vi "RangeXML_Flo.vi"() -> ()   [LabVIEW 2013]
panel:
  out "text":string
  out "LabVIEW Data 2":variant
  out "array":u16[](array[numeric])=[0, 0, 1, 1, 2, 2, 3, 3, 0, 0, 1, 1, 2, 2, 3, 3, 0, 0, 1, 1, 2, 2, 3, 3, 0, 0, 1, 1, 2, 2, 3, 3, 0, 0, 1, 1, 2, 2, 3, 3, 0, 0, 1, 1, 2, 2, 3, 3, 0, 0, 1, 1, 2, 2, 3, 3, 0, 0, 1, 1, 2, 2, 3, 3, 0, 0, 1, 1, 2, 2, 3, 3, 0, 0, 1, 1, 2, 2, 3, 3, 0, 0, 1, 1, 2, 2, 3, 3, 0, 0, 1, 1, 2, 2, 3, 3, 0, 0, 1, 1, 2, 2, 3, 3, 0, 0, 1, 1, 2, 2, 3, 3, 0, 0, 1, 1, 2, 2, 3, 3, 0, 0, 1, 1, 2, 2, 3, 3]
  in  "BoloRange_mV":T1={"Channel001"=0, "Channel002"=0, "Channel003"=1, "Channel004"=1, "Channel005"=2, "Channel006"=2, "Channel007"=3, "Channel008"=3, "Channel009"=0, "Channel010"=0, "Channel011"=1, "Channel012"=1, "Channel013"=2, "Channel014"=2, "Channel015"=3, "Channel016"=3, "Channel017"=0, "Channel018"=0, "Channel019"=1, "Channel020"=1, "Channel021"=2, "Channel022"=2, "Channel023"=3, "Channel024"=3, "Channel025"=0, "Channel026"=0, "Channel027"=1, "Channel028"=1, "Channel029"=2, "Channel030"=2, "Channel031"=3, "Channel032"=3, "Channel033"=0, "Channel034"=0, "Channel035"=1, "Channel036"=1, "Channel037"=2, "Channel038"=2, "Channel039"=3, "Channel040"=3, "Channel041"=0, "Channel042"=0, "Channel043"=1, "Channel044"=1, "Channel045"=2, "Channel046"=2, "Channel047"=3, "Channel048"=3, "Channel049"=0, "Channel050"=0, "Channel051"=1, "Channel052"=1, "Channel053"=2, "Channel054"=2, "Channel055"=3, "Channel056"=3, "Channel057"=0, "Channel058"=0, "Channel059"=1, "Channel060"=1, "Channel061"=2, "Channel062"=2, "Channel063"=3, "Channel064"=3, "Channel065"=0, "Channel066"=0, "Channel067"=1, "Channel068"=1, "Channel069"=2, "Channel070"=2, "Channel071"=3, "Channel072"=3, "Channel073"=0, "Channel074"=0, "Channel075"=1, "Channel076"=1, "Channel077"=2, "Channel078"=2, "Channel079"=3, "Channel080"=3, "Channel081"=0, "Channel082"=0, "Channel083"=1, "Channel084"=1, "Channel085"=2, "Channel086"=2, "Channel087"=3, "Channel088"=3, "Channel089"=0, "Channel090"=0, "Channel091"=1, "Channel092"=1, "Channel093"=2, "Channel094"=2, "Channel095"=3, "Channel096"=3, "Channel097"=0, "Channel098"=0, "Channel099"=1, "Channel100"=1, "Channel101"=2, "Channel102"=2, "Channel103"=3, "Channel104"=3, "Channel105"=0, "Channel106"=0, "Channel107"=1, "Channel108"=1, "Channel109"=2, "Channel110"=2, "Channel111"=3, "Channel112"=3, "Channel113"=0, "Channel114"=0, "Channel115"=1, "Channel116"=1, "Channel117"=2, "Channel118"=2, "Channel119"=3, "Channel120"=3, "Channel121"=0, "Channel122"=0, "Channel123"=1, "Channe124"=1, "Channel125"=2, "Channel126"=2, "Channel127"=3, "Channel128"=3} {"Channel128" items=["10", "20", "40", "80"]; "Channel127" items=["10", "20", "40", "80"]; "Channel126" items=["10", "20", "40", "80"]; "Channel125" items=["10", "20", "40", "80"]; "Channe124" items=["10", "20", "40", "80"]; "Channel123" items=["10", "20", "40", "80"]; "Channel122" items=["10", "20", "40", "80"]; "Channel121" items=["10", "20", "40", "80"]; "Channel120" items=["10", "20", "40", "80"]; "Channel119" items=["10", "20", "40", "80"]; "Channel118" items=["10", "20", "40", "80"]; "Channel117" items=["10", "20", "40", "80"]; "Channel116" items=["10", "20", "40", "80"]; "Channel115" items=["10", "20", "40", "80"]; "Channel114" items=["10", "20", "40", "80"]; "Channel113" items=["10", "20", "40", "80"]; "Channel112" items=["10", "20", "40", "80"]; "Channel111" items=["10", "20", "40", "80"]; "Channel110" items=["10", "20", "40", "80"]; "Channel109" items=["10", "20", "40", "80"]; "Channel108" items=["10", "20", "40", "80"]; "Channel107" items=["10", "20", "40", "80"]; "Channel106" items=["10", "20", "40", "80"]; "Channel105" items=["10", "20", "40", "80"]; "Channel104" items=["10", "20", "40", "80"]; "Channel103" items=["10", "20", "40", "80"]; "Channel102" items=["10", "20", "40", "80"]; "Channel101" items=["10", "20", "40", "80"]; "Channel100" items=["10", "20", "40", "80"]; "Channel099" items=["10", "20", "40", "80"]; "Channel098" items=["10", "20", "40", "80"]; "Channel097" items=["10", "20", "40", "80"]; "Channel096" items=["10", "20", "40", "80"]; "Channel095" items=["10", "20", "40", "80"]; "Channel094" items=["10", "20", "40", "80"]; "Channel093" items=["10", "20", "40", "80"]; "Channel092" items=["10", "20", "40", "80"]; "Channel091" items=["10", "20", "40", "80"]; "Channel090" items=["10", "20", "40", "80"]; "Channel089" items=["10", "20", "40", "80"]; "Channel088" items=["10", "20", "40", "80"]; "Channel087" items=["10", "20", "40", "80"]; "Channel086" items=["10", "20", "40", "80"]; "Channel085" items=["10", "20", "40", "80"]; "Channel084" items=["10", "20", "40", "80"]; "Channel083" items=["10", "20", "40", "80"]; "Channel082" items=["10", "20", "40", "80"]; "Channel081" items=["10", "20", "40", "80"]; "Channel080" items=["10", "20", "40", "80"]; "Channel079" items=["10", "20", "40", "80"]; "Channel078" items=["10", "20", "40", "80"]; "Channel077" items=["10", "20", "40", "80"]; "Channel076" items=["10", "20", "40", "80"]; "Channel075" items=["10", "20", "40", "80"]; "Channel074" items=["10", "20", "40", "80"]; "Channel073" items=["10", "20", "40", "80"]; "Channel072" items=["10", "20", "40", "80"]; "Channel071" items=["10", "20", "40", "80"]; "Channel070" items=["10", "20", "40", "80"]; "Channel069" items=["10", "20", "40", "80"]; "Channel068" items=["10", "20", "40", "80"]; "Channel067" items=["10", "20", "40", "80"]; "Channel066" items=["10", "20", "40", "80"]; "Channel065" items=["10", "20", "40", "80"]; "Channel064" items=["10", "20", "40", "80"]; "Channel063" items=["10", "20", "40", "80"]; "Channel062" items=["10", "20", "40", "80"]; "Channel061" items=["10", "20", "40", "80"]; "Channel060" items=["10", "20", "40", "80"]; "Channel059" items=["10", "20", "40", "80"]; "Channel058" items=["10", "20", "40", "80"]; "Channel057" items=["10", "20", "40", "80"]; "Channel056" items=["10", "20", "40", "80"]; "Channel055" items=["10", "20", "40", "80"]; "Channel054" items=["10", "20", "40", "80"]; "Channel053" items=["10", "20", "40", "80"]; "Channel052" items=["10", "20", "40", "80"]; "Channel051" items=["10", "20", "40", "80"]; "Channel050" items=["10", "20", "40", "80"]; "Channel049" items=["10", "20", "40", "80"]; "Channel048" items=["10", "20", "40", "80"]; "Channel047" items=["10", "20", "40", "80"]; "Channel046" items=["10", "20", "40", "80"]; "Channel045" items=["10", "20", "40", "80"]; "Channel044" items=["10", "20", "40", "80"]; "Channel043" items=["10", "20", "40", "80"]; "Channel042" items=["10", "20", "40", "80"]; "Channel041" items=["10", "20", "40", "80"]; "Channel040" items=["10", "20", "40", "80"]; "Channel039" items=["10", "20", "40", "80"]; "Channel038" items=["10", "20", "40", "80"]; "Channel037" items=["10", "20", "40", "80"]; "Channel036" items=["10", "20", "40", "80"]; "Channel035" items=["10", "20", "40", "80"]; "Channel034" items=["10", "20", "40", "80"]; "Channel033" items=["10", "20", "40", "80"]; "Channel032" items=["10", "20", "40", "80"]; "Channel031" items=["10", "20", "40", "80"]; "Channel030" items=["10", "20", "40", "80"]; "Channel029" items=["10", "20", "40", "80"]; "Channel028" items=["10", "20", "40", "80"]; "Channel027" items=["10", "20", "40", "80"]; "Channel026" items=["10", "20", "40", "80"]; "Channel025" items=["10", "20", "40", "80"]; "Channel024" items=["10", "20", "40", "80"]; "Channel023" items=["10", "20", "40", "80"]; "Channel022" items=["10", "20", "40", "80"]; "Channel021" items=["10", "20", "40", "80"]; "Channel020" items=["10", "20", "40", "80"]; "Channel019" items=["10", "20", "40", "80"]; "Channel018" items=["10", "20", "40", "80"]; "Channel017" items=["10", "20", "40", "80"]; "Channel016" items=["10", "20", "40", "80"]; "Channel015" items=["10", "20", "40", "80"]; "Channel014" items=["10", "20", "40", "80"]; "Channel013" items=["10", "20", "40", "80"]; "Channel012" items=["10", "20", "40", "80"]; "Channel011" items=["10", "20", "40", "80"]; "Channel010" items=["10", "20", "40", "80"]; "Channel009" items=["10", "20", "40", "80"]; "Channel008" items=["10", "20", "40", "80"]; "Channel007" items=["10", "20", "40", "80"]; "Channel006" items=["10", "20", "40", "80"]; "Channel005" items=["10", "20", "40", "80"]; "Channel004" items=["10", "20", "40", "80"]; "Channel003" items=["10", "20", "40", "80"]; "Channel002" items=["10", "20", "40", "80"]; "Channel001" items=["10", "20", "40", "80"]}
  out "LabVIEW Data":variant=variant(cluster{"Channel001":u16, "Channel002":u16, "Channel003":u16, "Channel004":u16, "Channel005":u16, "Channel006":u16, "Channel007":u16, "Channel008":u16, "Channel009":u16, "Channel010 ":u16, "Channel011":u16, "Channel012":u16, "Channel013 ":u16, "Channel014":u16, "Channel015":u16, "Channel016":u16, "Channel017":u16, "Channel018 ":u16, "Channel019":u16, "Channel020":u16, "Channel021":u16, "Channel022":u16, "Channel023":u16, "Channel024":u16, "Channel025":u16, "Channel026":u16, "Channel027":u16, "Channel028":u16, "Channel029":u16, "Channel030":u16, "Channel031":u16, "Channel032":u16, "Channel033":u16, "Channel034":u16, "Channel035":u16, "Channel036":u16, "Channel037":u16, "Channel038":u16, "Channel039":u16, "Channel040":u16, "Channel041":u16, "Channel042":u16, "Channel043 ":u16, "Channel044":u16, "Channel045 ":u16, "Channel046":u16, "Channel047":u16, "Channel048":u16, "Channel049":u16, "Channel050 ":u16, "Channel051":u16, "Channel052":u16, "Channel053":u16, "Channel054":u16, "Channel55":u16, "Channel56":u16, "Channel57":u16, "Channel58":u16, "Channel59":u16, "Channe60":u16, "Channel61":u16, "Channel62":u16, "Channe63":u16, "Channel64":u16, "Channel65":u16, "Channel66":u16, "Channel67":u16, "Channel68":u16, "Channel69":u16, "Channel70":u16, "Channel71":u16, "Channel72":u16, "Channel73":u16, "Channel74 ":u16, "Channel75":u16, "Channe76":u16, "Channel77":u16, "Channel78":u16, "Channel79":u16, "Channel80":u16, "Channel81":u16, "Channel82 ":u16, "Channel83":u16, "Channel84":u16, "Channel85":u16, "Channel86":u16, "Channel87":u16, "Channel88":u16, "Channel89":u16, "Channel90":u16, "Channel91":u16, "Channe92":u16, "Channel93":u16, "Channel94":u16, "Channe95":u16, "Channel96":u16, "Channel97":u16, "Channel98":u16, "Channel99":u16, "Channel36 2":u16, "Channel37 2":u16, "Channel38 2":u16, "Channel39 2":u16, "Channel40 2":u16, "Channel41 2":u16, "Channel42 2":u16, "Channel43  2":u16, "Channe44 2":u16, "Channel45  2":u16, "Channel46 2":u16, "Channel47 2":u16, "Channel48 2":u16, "Channel113":u16, "Channel114":u16, "Channel115":u16, "Channel116":u16, "Channel117":u16, "Channel118":u16, "Channel119":u16, "Channel120":u16, "Channel121":u16, "Channel122":u16, "Channel123":u16, "Channe124":u16, "Channel125":u16, "Channel126":u16, "Channel127":u16, "Channel128":u16} {"Channel001"=0, "Channel002"=0, "Channel003"=1, "Channel004"=1, "Channel005"=2, "Channel006"=2, "Channel007"=3, "Channel008"=3, "Channel009"=0, "Channel010 "=0, "Channel011"=1, "Channel012"=1, "Channel013 "=2, "Channel014"=2, "Channel015"=3, "Channel016"=3, "Channel017"=0, "Channel018 "=0, "Channel019"=1, "Channel020"=1, "Channel021"=2, "Channel022"=2, "Channel023"=3, "Channel024"=3, "Channel025"=0, "Channel026"=0, "Channel027"=1, "Channel028"=1, "Channel029"=2, "Channel030"=2, "Channel031"=3, "Channel032"=3, "Channel033"=0, "Channel034"=0, "Channel035"=1, "Channel036"=1, "Channel037"=2, "Channel038"=2, "Channel039"=3, "Channel040"=3, "Channel041"=0, "Channel042"=0, "Channel043 "=1, "Channel044"=1, "Channel045 "=2, "Channel046"=2, "Channel047"=3, "Channel048"=3, "Channel049"=0, "Channel050 "=0, "Channel051"=1, "Channel052"=1, "Channel053"=2, "Channel054"=2, "Channel55"=3, "Channel56"=3, "Channel57"=0, "Channel58"=0, "Channel59"=1, "Channe60"=1, "Channel61"=2, "Channel62"=2, "Channe63"=3, "Channel64"=3, "Channel65"=0, "Channel66"=0, "Channel67"=1, "Channel68"=1, "Channel69"=2, "Channel70"=2, "Channel71"=3, "Channel72"=3, "Channel73"=0, "Channel74 "=0, "Channel75"=1, "Channe76"=1, "Channel77"=2, "Channel78"=2, "Channel79"=3, "Channel80"=3, "Channel81"=0, "Channel82 "=0, "Channel83"=1, "Channel84"=1, "Channel85"=2, "Channel86"=2, "Channel87"=3, "Channel88"=3, "Channel89"=0, "Channel90"=0, "Channel91"=1, "Channe92"=1, "Channel93"=2, "Channel94"=2, "Channe95"=3, "Channel96"=3, "Channel97"=0, "Channel98"=0, "Channel99"=1, "Channel36 2"=1, "Channel37 2"=2, "Channel38 2"=2, "Channel39 2"=3, "Channel40 2"=3, "Channel41 2"=0, "Channel42 2"=0, "Channel43  2"=1, "Channe44 2"=1, "Channel45  2"=2, "Channel46 2"=2, "Channel47 2"=3, "Channel48 2"=3, "Channel113"=0, "Channel114"=0, "Channel115"=1, "Channel116"=1, "Channel117"=2, "Channel118"=2, "Channel119"=3, "Channel120"=3, "Channel121"=0, "Channel122"=0, "Channel123"=1, "Channe124"=1, "Channel125"=2, "Channel126"=2, "Channel127"=3, "Channel128"=3})
  out "XML String":string="<BoloRange_mV>\r\n  <Channel001>0</Channel001>\r\n  <Channel002>0</Channel002>\r\n  <Channel003>1</Channel003>\r\n  <Channel004>1</Channel004>\r\n  <Channel005>2</Channel005>\r\n  <Channel006>2</Channel006>\r\n  <Channel007>3</Channel007>\r\n  <Channel008>3</Channel008>\r\n  <Channel009>0</Channel009>\r\n  <Channel010_>0</Channel010_>\r\n  <Channel011>1</Channel011>\r\n  <Channel012>1</Channel012>\r\n  <Channel013_>2</Channel013_>\r\n  <Channel014>2</Channel014>\r\n  <Channel015>3</Channel015>\r\n  <Channel016>3</Channel016>\r\n  <Channel017>0</Channel017>\r\n  <Channel018_>0</Channel018_>\r\n  <Channel019>1</Channel019>\r\n  <Channel020>1</Channel020>\r\n  <Channel021>2</Channel021>\r\n  <Channel022>2</Channel022>\r\n  <Channel023>3</Channel023>\r\n  <Channel024>3</Channel024>\r\n  <Channel025>0</Channel025>\r\n  <Channel026>0</Channel026>\r\n  <Channel027>1</Channel027>\r\n  <Channel028>1</Channel028>\r\n  <Channel029>2</Channel029>\r\n  <Channel030>2</Channel030>\r\n  <Channel031>3</Channel031>\r\n  <Channel032>3</Channel032>\r\n  <Channel033>0</Channel033>\r\n  <Channel034>0</Channel034>\r\n  <Channel035>1</Channel035>\r\n  <Channel036>1</Channel036>\r\n  <Channel037>2</Channel037>\r\n  <Channel038>2</Channel038>\r\n  <Channel039>3</Channel039>\r\n  <Channel040>3</Channel040>\r\n  <Channel041>0</Channel041>\r\n  <Channel042>0</Channel042>\r\n  <Channel043_>1</Channel043_>\r\n  <Channel044>1</Channel044>\r\n  <Channel045_>2</Channel045_>\r\n  <Channel046>2</Channel046>\r\n  <Channel047>3</Channel047>\r\n  <Channel048>3</Channel048>\r\n  <Channel049>0</Channel049>\r\n  <Channel050_>0</Channel050_>\r\n  <Channel051>1</Channel051>\r\n  <Channel052>1</Channel052>\r\n  <Channel053>2</Channel053>\r\n  <Channel054>2</Channel054>\r\n  <Channel055>3</Channel055>\r\n  <Channel056>3</Channel056>\r\n  <Channel057>0</Channel057>\r\n  <Channel058>0</Channel058>\r\n  <Channel059>1</Channel059>\r\n  <Channe60>1</Channe60>\r\n  <Channel061>2</Channel061>\r\n  <Channel062>2</Channel062>\r\n  <Channe63>3</Channe63>\r\n  <Channel064>3</Channel064>\r\n  <Channel065>0</Channel065>\r\n  <Channel066>0</Channel066>\r\n  <Channel067>1</Channel067>\r\n  <Channel068>1</Channel068>\r\n  <Channel069>2</Channel069>\r\n  <Channel070>2</Channel070>\r\n  <Channel071>3</Channel071>\r\n  <Channel072>3</Channel072>\r\n  <Channel073>0</Channel073>\r\n  <Channel074_>0</Channel074_>\r\n  <Channel075>1</Channel075>\r\n  <Channe76>1</Channe76>\r\n  <Channel077>2</Channel077>\r\n  <Channel078>2</Channel078>\r\n  <Channel079>3</Channel079>\r\n  <Channel080>3</Channel080>\r\n  <Channel081>0</Channel081>\r\n  <Channel082_>0</Channel082_>\r\n  <Channel083>1</Channel083>\r\n  <Channel084>1</Channel084>\r\n  <Channel085>2</Channel085>\r\n  <Channel086>2</Channel086>\r\n  <Channel087>3</Channel087>\r\n  <Channel088>3</Channel088>\r\n  <Channel089>0</Channel089>\r\n  <Channel090>0</Channel090>\r\n  <Channel091>1</Channel091>\r\n  <Channe92>1</Channe92>\r\n  <Channel093>2</Channel093>\r\n  <Channel094>2</Channel094>\r\n  <Channe95>3</Channe95>\r\n  <Channel096>3</Channel096>\r\n  <Channel097>0</Channel097>\r\n  <Channel098>0</Channel098>\r\n  <Channel099>1</Channel099>\r\n  <Channel36_2>1</Channel36_2>\r\n  <Channel37_2>2</Channel37_2>\r\n  <Channel38_2>2</Channel38_2>\r\n  <Channel39_2>3</Channel39_2>\r\n  <Channel40_2>3</Channel40_2>\r\n  <Channel41_2>0</Channel41_2>\r\n  <Channel42_2>0</Channel42_2>\r\n  <Channel43__2>1</Channel43__2>\r\n  <Channe44_2>1</Channe44_2>\r\n  <Channel45__2>2</Channel45__2>\r\n  <Channel46_2>2</Channel46_2>\r\n  <Channel47_2>3</Channel47_2>\r\n  <Channel48_2>3</Channel48_2>\r\n  <Channel113>0</Channel113>\r\n  <Channel114>0</Channel114>\r\n  <Channel115>1</Channel115>\r\n  <Channel116>1</Channel116>\r\n  <Channel117>2</Channel117>\r\n  <Channel118>2</Channel118>\r\n  <Channel119>3</Channel119>\r\n  <Channel120>3</Channel120>\r\n  <Channel121>0</Channel121>\r\n  <Channel122>0</Channel122>\r\n  <Channel123>1</Channel123>\r\n  <Channe124>1</Channe124>\r\n  <Channel125>2</Channel125>\r\n  <Channel126>2</Channel126>\r\n  <Channel127>3</Channel127>\r\n  <Channel128>3</Channel128>\r\n</BoloRange_mV>"
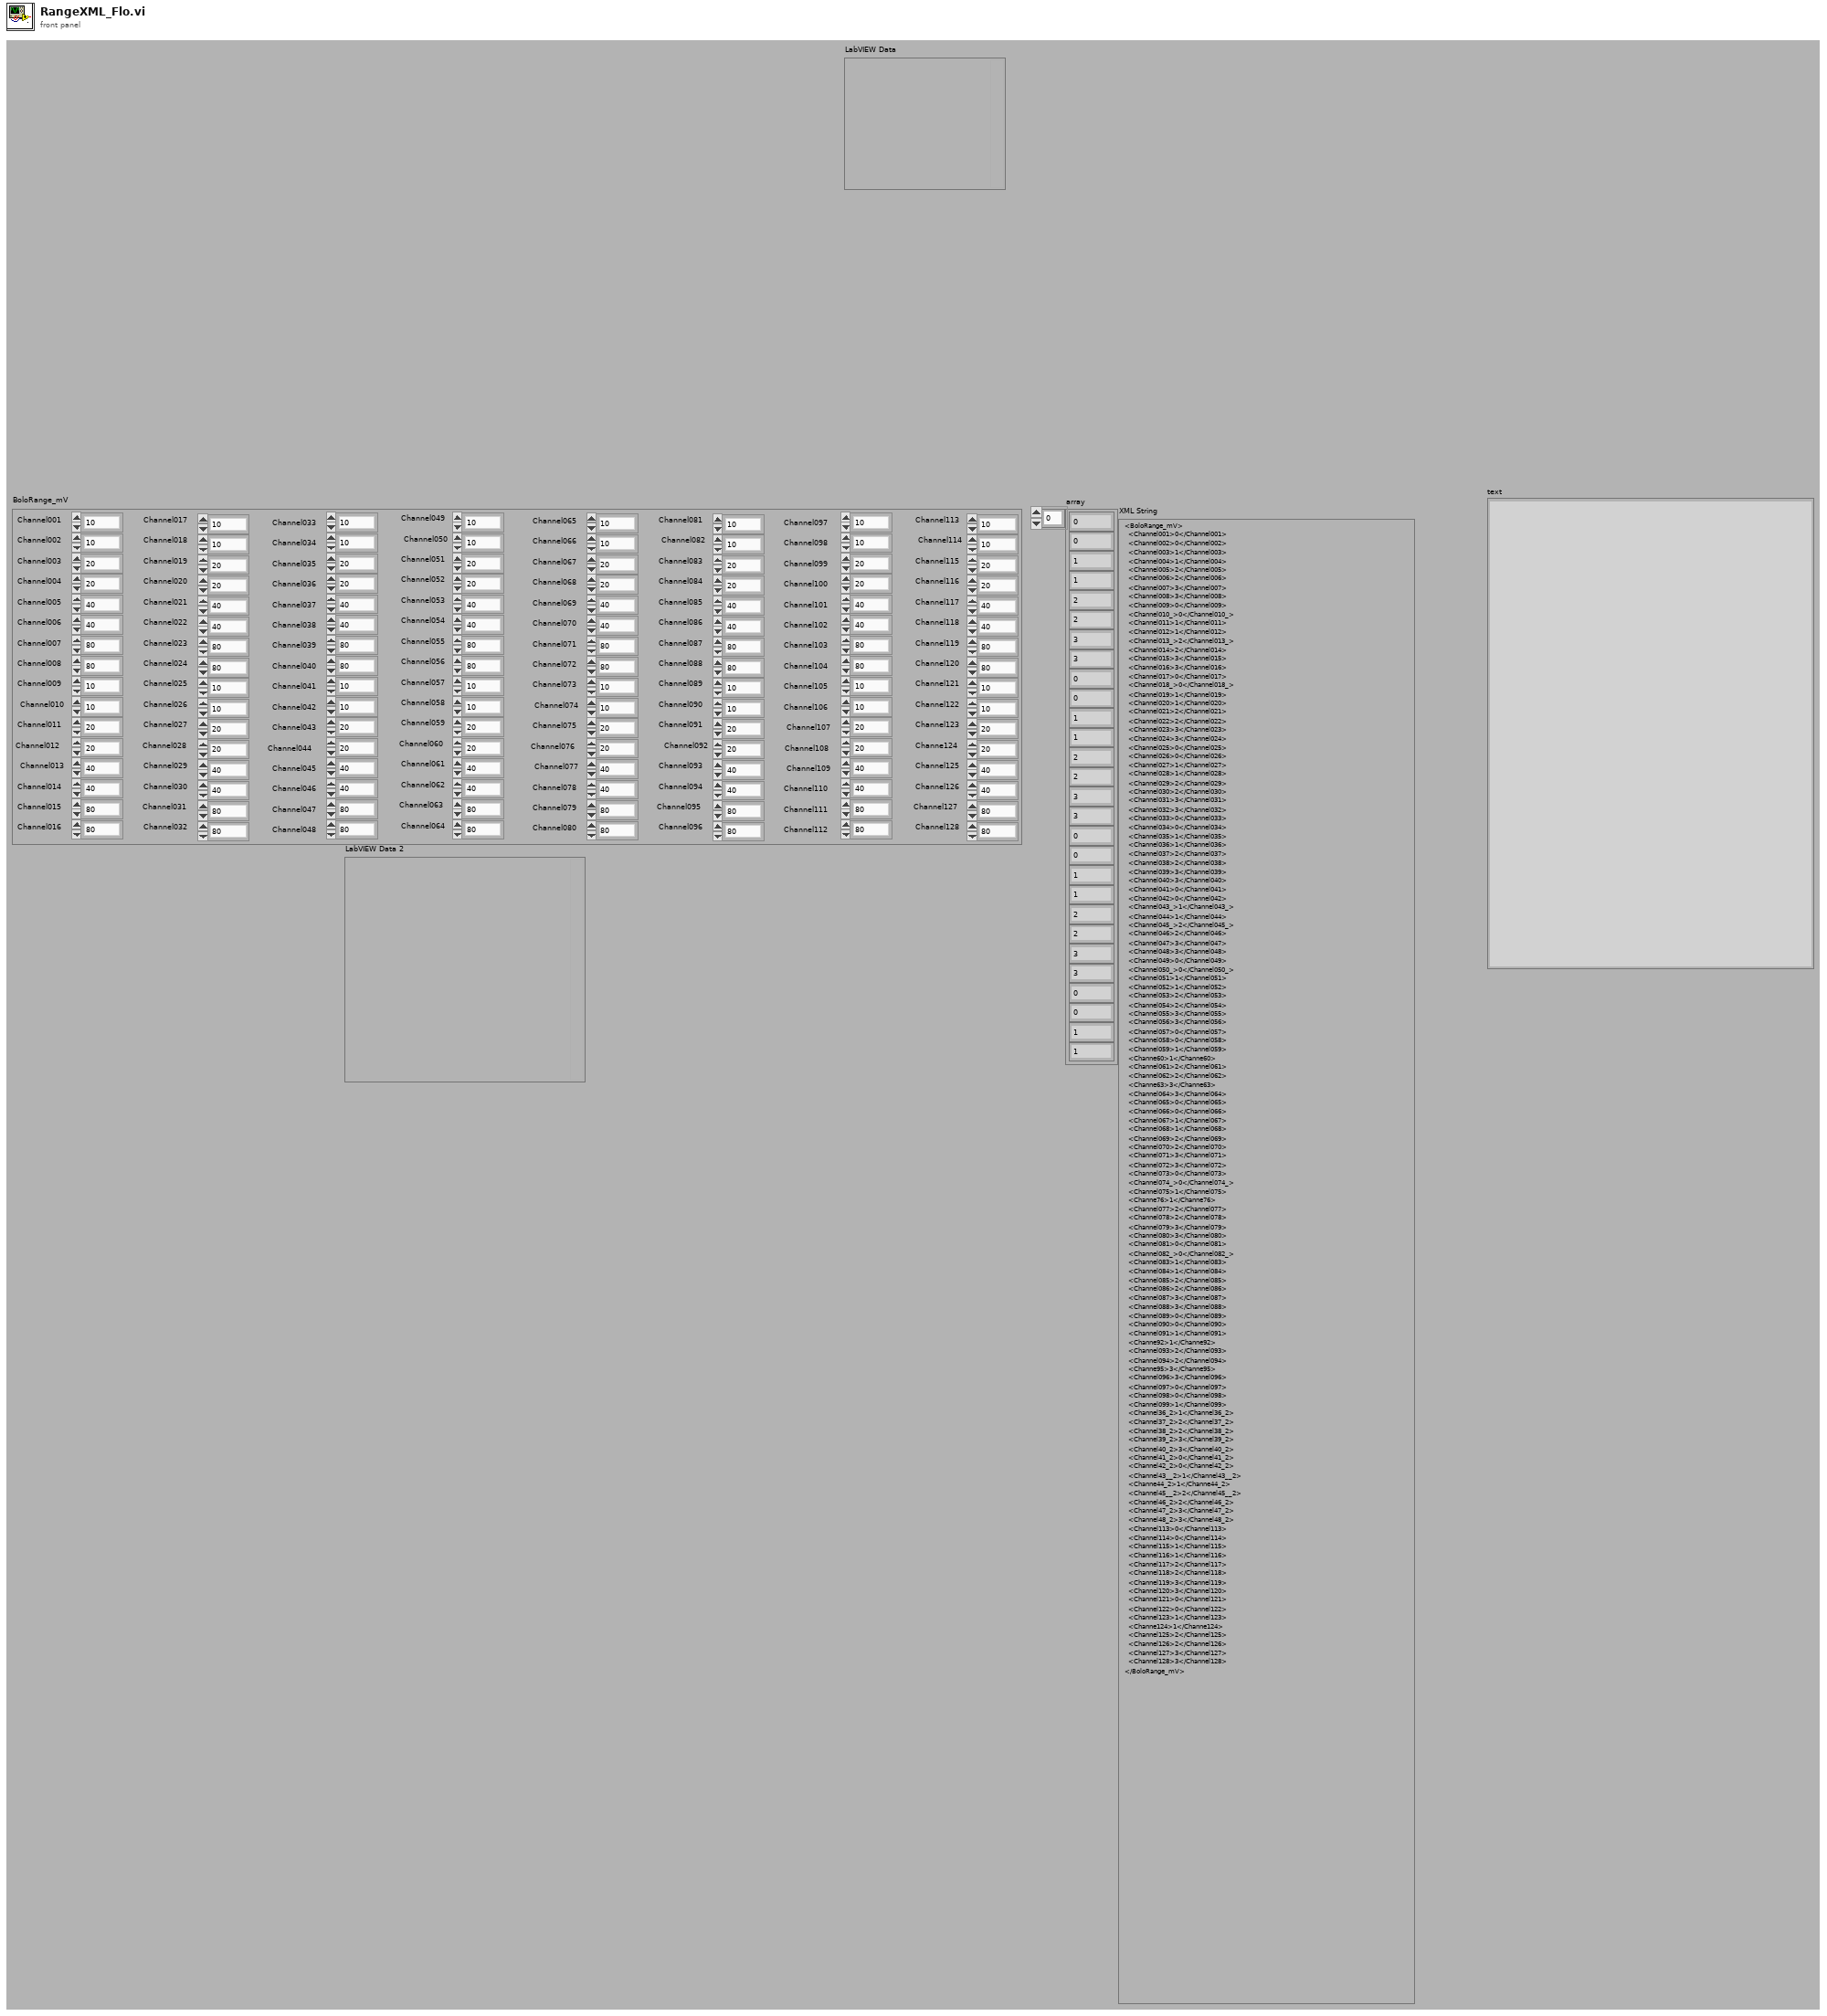
[diagram p1: front panel]
types:
  T1 = cluster{"Channel001":u16, "Channel002":u16, "Channel003":u16, "Channel004":u16, "Channel005":u16, "Channel006":u16, "Channel007":u16, "Channel008":u16, "Channel009":u16, "Channel010":u16, "Channel011":u16, "Channel012":u16, "Channel013":u16, "Channel014":u16, "Channel015":u16, "Channel016":u16, "Channel017":u16, "Channel018":u16, "Channel019":u16, "Channel020":u16, "Channel021":u16, "Channel022":u16, "Channel023":u16, "Channel024":u16, "Channel025":u16, "Channel026":u16, "Channel027":u16, "Channel028":u16, "Channel029":u16, "Channel030":u16, "Channel031":u16, "Channel032":u16, "Channel033":u16, "Channel034":u16, "Channel035":u16, "Channel036":u16, "Channel037":u16, "Channel038":u16, "Channel039":u16, "Channel040":u16, "Channel041":u16, "Channel042":u16, "Channel043":u16, "Channel044":u16, "Channel045":u16, "Channel046":u16, "Channel047":u16, "Channel048":u16, "Channel049":u16, "Channel050":u16, "Channel051":u16, "Channel052":u16, "Channel053":u16, "Channel054":u16, "Channel055":u16, "Channel056":u16, "Channel057":u16, "Channel058":u16, "Channel059":u16, "Channel060":u16, "Channel061":u16, "Channel062":u16, "Channel063":u16, "Channel064":u16, "Channel065":u16, "Channel066":u16, "Channel067":u16, "Channel068":u16, "Channel069":u16, "Channel070":u16, "Channel071":u16, "Channel072":u16, "Channel073":u16, "Channel074":u16, "Channel075":u16, "Channel076":u16, "Channel077":u16, "Channel078":u16, "Channel079":u16, "Channel080":u16, "Channel081":u16, "Channel082":u16, "Channel083":u16, "Channel084":u16, "Channel085":u16, "Channel086":u16, "Channel087":u16, "Channel088":u16, "Channel089":u16, "Channel090":u16, "Channel091":u16, "Channel092":u16, "Channel093":u16, "Channel094":u16, "Channel095":u16, "Channel096":u16, "Channel097":u16, "Channel098":u16, "Channel099":u16, "Channel100":u16, "Channel101":u16, "Channel102":u16, "Channel103":u16, "Channel104":u16, "Channel105":u16, "Channel106":u16, "Channel107":u16, "Channel108":u16, "Channel109":u16, "Channel110":u16, "Channel111":u16, "Channel112":u16, "Channel113":u16, "Channel114":u16, "Channel115":u16, "Channel116":u16, "Channel117":u16, "Channel118":u16, "Channel119":u16, "Channel120":u16, "Channel121":u16, "Channel122":u16, "Channel123":u16, "Channe124":u16, "Channel125":u16, "Channel126":u16, "Channel127":u16, "Channel128":u16}
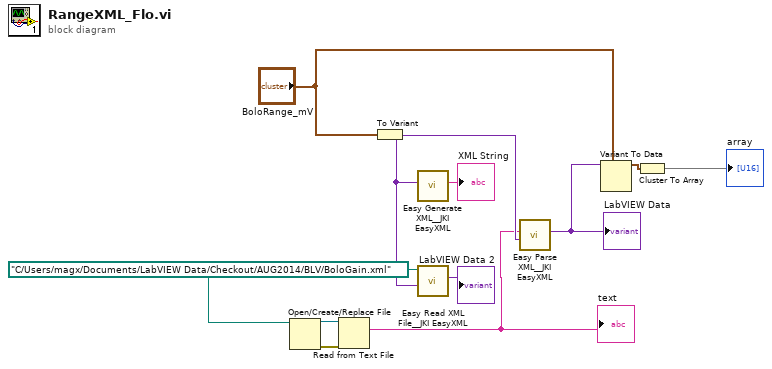
[diagram p0: block diagram]
diagram:
  w5 = path "C:/Users/magx/Documents/LabVIEW Data/Checkout/AUG2014/BLV/BoloGain.xml" ("XML File Path")
  n1 = Open/Create/Replace File(file path (use dialog)=w5) -> (refnum out=w3:refnum<file>, error out=w4:errorcluster)  [unwired: 1 in, 5 out]
  n2 = Read from Text File(file (use dialog)=w3, error in=w4) -> (text=w1:string)  [unwired: 5 out]
  "text" <- w1
  n3 = To Variant(anything="BoloRange_mV") -> (Variant=w2:variant)
  n4 = call <vilib>:"Easy Generate XML__JKI EasyXML.vi"("LabVIEW Data"=w2) -> ("XML String"=→"XML String":string)  [unwired: 1 in, 9 out]
  n5 = call <vilib>:"Easy Read XML File__JKI EasyXML.vi"("LabVIEW Data (Type)"=w2, "XML File Path"=w5) -> ("LabVIEW Data"=→"LabVIEW Data 2":variant)  [unwired: 1 in, 8 out]
  n6 = call <vilib>:"Easy Parse XML__JKI EasyXML.vi"("LabVIEW Data (Type)"=w2, "XML String"=w1) -> ("LabVIEW Data"=w10:variant)  [unwired: 1 in, 8 out]
  "LabVIEW Data" <- w10
  n7 = Variant To Data(type="BoloRange_mV", Variant=w10) -> (data=w9:T1)  [unwired: 1 in, 1 out]
  n8 = Cluster To Array(cluster=w9) -> (array=→"array":u16[])
